vi "IRIS_set_Position.vi"(8 "error in (no error)":errorcluster, 10 "Channel parsed command info":T1, 11 "IRIS in":refnum<class "ISSI_Iris.lvclass">) -> (0 "error out":errorcluster, 2 "new commands":string, 3 "MKS4000b out":refnum<class "ISSI_Iris.lvclass">)   [LabVIEW 2020, in "ISSI_Iris.lvclass"]
uses:
  ISSI_Iris.lvclass
  Shared/Device Driver/channel parsed cmd cluster.ctl
  ISSI_Iris.lvclass/ISSI_Iris.ctl
  shared/CompressAndUpdate(Poly)/CompressAndUpdate(Numeric).vi
panel:
  out "data out":string
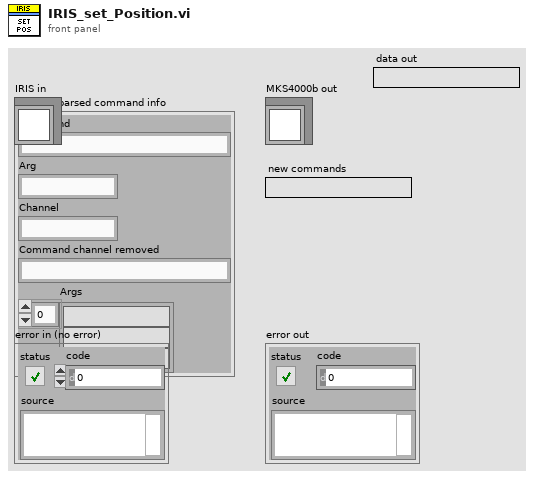
[diagram p1: front panel]
types:
  T1 = typedef "channel parsed cmd cluster.ctl" = cluster{"Command":string, "Arg":string, "Channel":string, "Command channel removed":string, "Args":string[]}
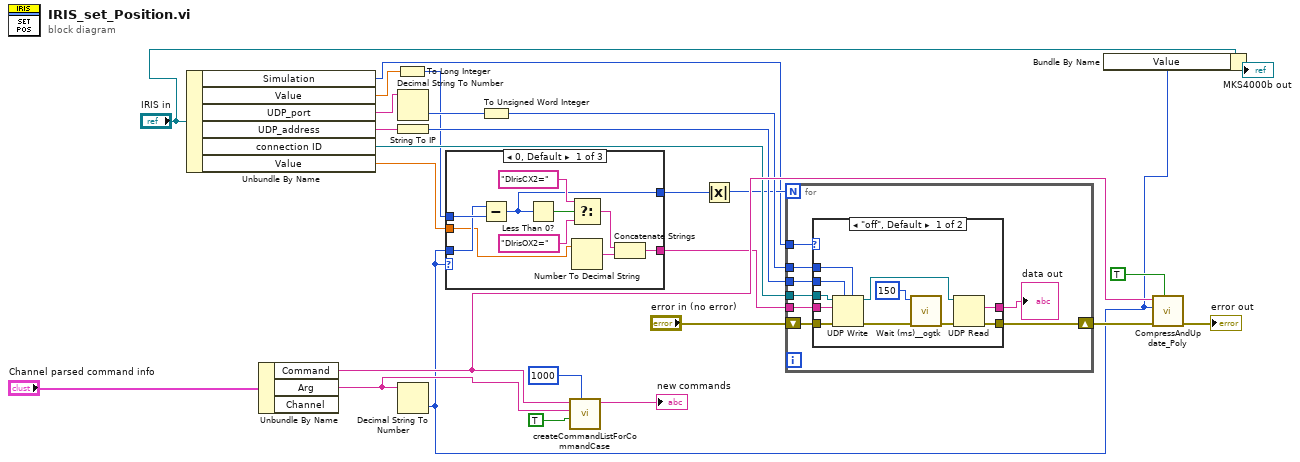
[diagram p0: block diagram]
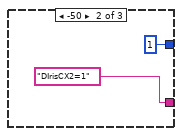
[diagram p2: hidden frame]
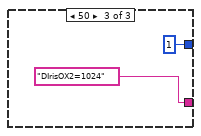
[diagram p3: hidden frame]
diagram:
  n1 = Unbundle By Name("IRIS in") -> ("Simulation"=w8:enum16{"off", "on"}, "Value"=w10:dbl, "UDP_port"=w15:string, "UDP_address"=w17:string, "connection ID"=w16:refnum<k16>, "Value"=w7:dbl)
  n2 = Unbundle By Name("Channel parsed command info") -> ("Command"=w26:string, "Arg"=w25:string)  [unwired: 1 out]
  n3 = To Long Integer(number=w10) -> (32bit integer=w9:i32)
  n4 = Decimal String To Number(string=w15) -> (number=w14:i32)  [unwired: 2 in, 1 out]
  n5 = String To IP(1:w17) -> (0:w18:u32)
  n6 = Decimal String To Number(string=w25) -> (number=w1:i32)  [unwired: 2 in, 1 out]
  n7 = case shown="0, Default" w1 {
    tunnel: [w33 1 1] -> w12
    tunnel: w9 -> [w32 _ _]
    tunnel: w1 -> [w31 _ _]
    tunnel: w7 -> [w29 _ _]
    tunnel: [w27 "DIrisCX2=1" ("string") "DIrisOX2=1024" ("string")] -> w6
    frame 0, Default {
      n8 = Subtract(x=w31, y=w32) -> (x-y=w33:i32)
      n9 = Less Than 0?(x=w33) -> (x < 0?=w36:bool)
      n10 = Select(t="DIrisCX2=" ("string"), s=w36, f="DIrisOX2=" ("string")) -> (s? t:f=w28:string)
      n11 = Number To Decimal String(number=w29) -> (decimal integer string=w30:string)  [unwired: 1 in]
      n12 = Concatenate Strings(w28, w30) -> (w27:string)
    }
    frame -50 {
    }
    frame 50 {
    }
  }
  n13 = To Unsigned Word Integer(number=w14) -> (unsigned 16bit integer=w13:u16)
  n14 = call "createCommandListForCommandCase.vi"("timeout (optional)"=1000, "immediate Check (only once)"=TRUE, "setvalue"=w25, "command"=w26) -> ("new commands"=→"new commands":string)  [unwired: 7 in]
  n15 = Absolute Value(x=w12) -> (abs(x)=w11:i32)
  n16 = for {
    N: w11 -> [_]
    tunnel: w6 -> [w48]
    tunnel: w18 -> [w46]
    tunnel: w16 -> [w45]
    tunnel: w13 -> [w44]
    shift-right: [w43] -> w19
    shift-left: "error in (no error)" -> [w47]
    tunnel: w8 -> [w41]
    n17 = case shown="\"off\", Default" w41 {
      tunnel: w48 -> [w59 w61]
      tunnel: w47 -> [w58 w60]
      tunnel: w46 -> [w57 _]
      tunnel: w45 -> [w56 _]
      tunnel: w44 -> [w55 _]
      tunnel: [w50 w60] -> w43
      tunnel: [w49 w61] -> w42
      frame "off", Default {
        n18 = UDP Write(address=w57, port or service name=w55, connection ID=w56, data in=w59, 8:w58) -> (error out=w54:errorcluster, 3:w51:refnum<k16>)  [unwired: 1 in]
        n19 = call <userlib>:"Wait (ms)__ogtk.vi"("error in (no error)"=w54, "milliseconds to wait"=u32 150) -> ("error out"=w52:errorcluster)  [unwired: 8 in, 1 out]
        n20 = UDP Read(connection ID=w51, 8:w52) -> (data out=w49:string, error out=w50:errorcluster)  [unwired: 2 in, 3 out]
      }
      frame "on" {
      }
    }
    "data out" <- w42
  }
  n21 = Bundle By Name(cluster="IRIS in", "Value"=w1) -> (→"MKS4000b out":refnum<class "ISSI_Iris.lvclass">)
  n22 = call-poly "CompressAndUpdate_Poly.vi"("force CVT update (false)"=TRUE ("force CVT update"), "error in"=w19, "Numeric"=w1, "command or variable name"=w26) -> ("error out"=→"error out":errorcluster)  [unwired: 7 in]
